vi "SDCP - Standard Message Frames Editor - Load Excel File.vi"(2 "error in (no error)":errorcluster, 3 "Excel File Path":path=path "E:/Projects/System Diagnostics and Control Protocol/SDCP_LabVIEW/Parameter Files/Motion Processing Board - Standard Message Frame List.csv") -> (0 "error out":errorcluster, 1 "Parameters":T2(array[cluster]))   [LabVIEW 2020]
uses:
  Typedefs/SDCP - Standard Message Frames Editor - Parameter cluster.ctl
  <vilib>/Utility/NIReport.llb/Report Type.ctl
  <vilib>/addons/_office/excel.llb/Excel Get Data ([str]).vi
  <vilib>/Utility/NIReport.llb/NI_report.lvclass
  <vilib>/Utility/NIReport.llb/NI_ReportGenerationCore.lvlib
  <vilib>/Utility/NIReport.llb/Excel/NI_Excel.lvclass
  <vilib>/addons/_office/NI_ReportGenerationToolkit.lvlib
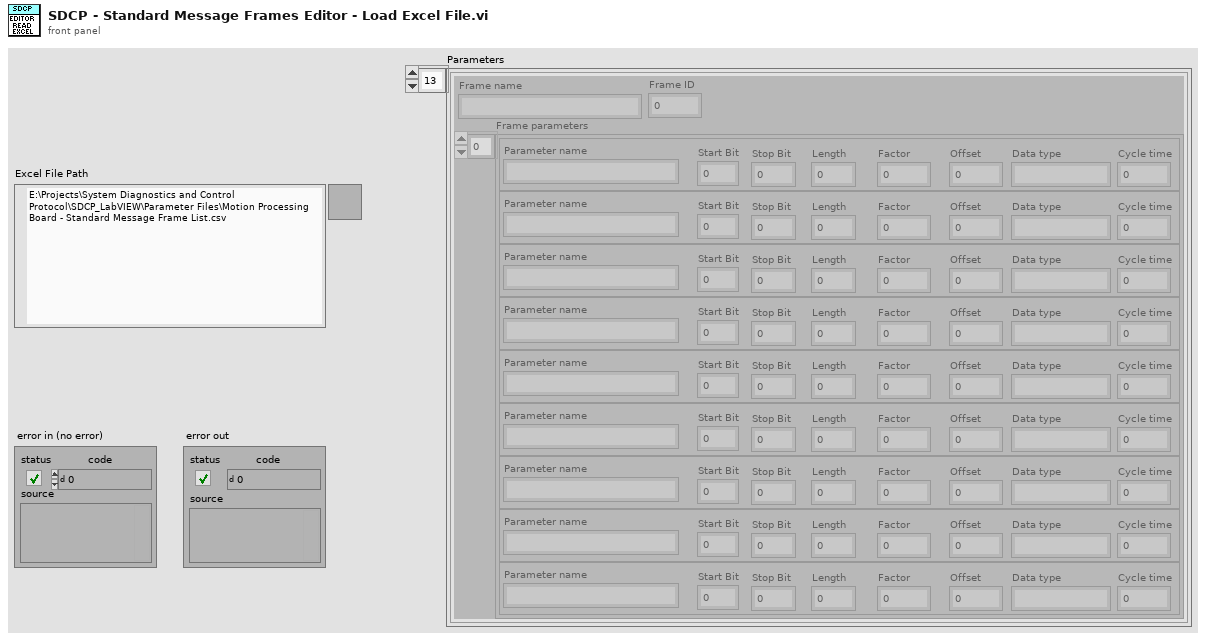
[diagram p1: front panel]
types:
  T1 = typedef "SDCP - Standard Message Frames Editor - Parameter cluster.ctl" = cluster{"Parameter name":string, "Start Bit":i32, "Stop Bit":i32, "Length":i32, "Factor":dbl, "Offset":dbl, "Data type":string, "Cycle time":dbl}
  T2 = cluster{"Frame name":string, "Frame ID":i32, "Frame parameters":T1[]}[]
  T3 = typedef "NI_ReportGenerationCore.lvlib/Report Type.ctl" = enum16{"HTML", "Word", "Excel"}
  T4 = enum16{"maximized", "minimized", "normal", "no change"}
  T5 = cluster{"Frame name":string, "Frame ID":i32, "Frame parameters":T1[]}
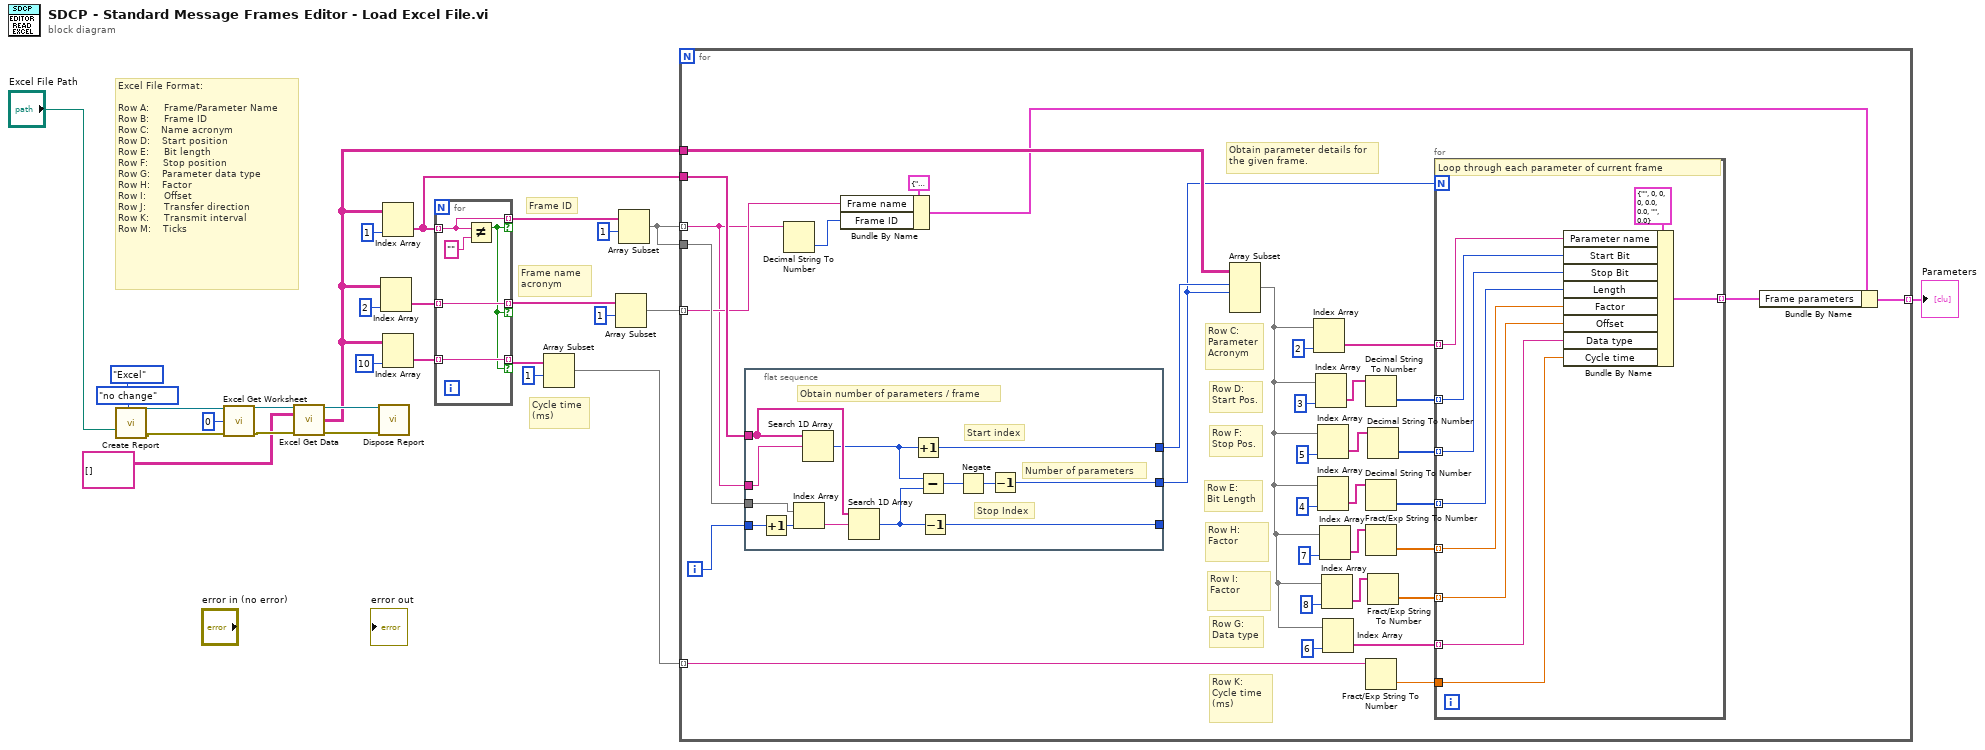
[diagram p0: block diagram]
diagram:
  # "Cycle time\n(ms)"
  # "Frame name \nacronym"
  # "Frame ID"
  # "Excel File Format: \n\nRow A:     Frame/Parameter Name\nRow B:     Frame ID\nRow C:    Name acronym\nRow D:    Start position\nRow E:     Bit length\nRow F:     Stop position\nRow G:    Parameter data type\nRow H:    Factor\nRow I:      Offset\nRow J:      Transfer direction\nRow K:     Transmit interval\nRow M:    Ticks"
  n1 = call <vilib>:"Create Report.vi"("window state (normal)"=T4."no change", "report type"=Report_Type."Excel", "template (empty)"="Excel File Path") -> ("report out"=w24:refnum<class "NI_report.lvclass">, "error out"=w25:errorcluster)  [unwired: 11 in]
  n2 = call <vilib>:"Excel Get Worksheet.vi"("report in"=w24, "worksheet index (0)"=0, "error in (no error)"=w25) -> ("report out"=w22:refnum<class "NI_report.lvclass">, "error out"=w21:errorcluster)  [unwired: 11 in]
  n3 = call-poly <vilib>:"Excel Get Data.vi"("report in"=w22, "data type"=string[][] [], "error in (no error)"=w21) -> ("report out"=w12:refnum<class "NI_report.lvclass">, "data"=w5:string[][], "error out"=w11:errorcluster)  [unwired: 10 in]
  n4 = call-dynamic "Dispose Report.vi"("report in"=w12, "error in (no error)"=w11) -> ()  [unwired: 13 in, 1 out]
  n5 = Index Array(array=w5, index (col)=2 ("disabled index (col)")) -> (element=w15:string[])  [unwired: 1 in]
  n6 = Index Array(array=w5, index (col)=1 ("disabled index (col)")) -> (element=w9:string[])  [unwired: 1 in]
  n7 = Index Array(array=w5, index (col)=10 ("disabled index (col)")) -> (element=w4:string[])  [unwired: 1 in]
  n8 = for {
    tunnel: w9 -> [w32] mode=indexing
    tunnel: [w32] -> w18 mode=indexing if=w29
    tunnel: w15 -> [w31] mode=indexing
    tunnel: [w31] -> w13 mode=indexing if=w29
    tunnel: w4 -> [w30] mode=indexing
    tunnel: [w30] -> w2 mode=indexing if=w29
    n9 = Not Equal?(x=w32, y="") -> (x != y?=w29:bool)
  }
  n10 = Array Subset(array=w2, index=1) -> (w1:string[])  [unwired: 1 in]
  n11 = Array Subset(array=w13, index=1) -> (w10:string[])  [unwired: 1 in]
  n12 = Array Subset(array=w18, index=1) -> (w8:string[])  [unwired: 1 in]
  n13 = for {
    tunnel: w8 -> [w63] mode=indexing
    tunnel: w10 -> [w64] mode=indexing
    tunnel: w5 -> [w61]
    tunnel: w9 -> [w66]
    tunnel: w8 -> [w68]
    tunnel: [w39] -> w7 mode=indexing
    tunnel: w1 -> [w34] mode=indexing
    i -> [w67]
    # "Row G:\nData type"
    # "Row K:\nCycle time\n(ms)"
    # "Row I:\nFactor"
    # "Row H:\nFactor"
    # "Row E:\nBit Length"
    # "Row F: \nStop Pos."
    # "Row D:\nStart Pos."
    # "Row C: \nParameter\nAcronym"
    # "Obtain parameter details for\nthe given frame."
    n14 = flat-sequence {
      tunnel: w63 -> [w91]
      tunnel: w68 -> [w90]
      tunnel: w67 -> [w89]
      tunnel: w66 -> [w87]
      tunnel: [w83] -> w59
      tunnel: [w81] -> w60
      tunnel: [w79] -> _
      frame #0 {
        # "Stop Index"
        # "Number of parameters"
        # "Start index"
        # "Obtain number of parameters / frame"
        n15 = Increment(x=w89) -> (x+1=w88:i32)
        n16 = Index Array(array=w90, index=w88) -> (element=w85:string)
        n17 = Search 1D Array(1D array=w87, element=w91) -> (index of element=w82:i32)  [unwired: 1 in]
        n18 = Search 1D Array(1D array=w87, element=w85) -> (index of element=w80:i32)  [unwired: 1 in]
        n19 = Increment(x=w82) -> (x+1=w81:i32)
        n20 = Subtract(x=w82, y=w80) -> (x-y=w86:i32)
        n21 = Decrement(x=w80) -> (x-1=w79:i32)
        n22 = Negate(x=w86) -> (-x=w84:i32)
        n23 = Decrement(x=w84) -> (x-1=w83:i32)
      }
    }
    n24 = Decimal String To Number(string=w63) -> (number=w62:i32)  [unwired: 2 in, 1 out]
    n25 = Bundle By Name(cluster=T5 {"Frame name"="", "Frame ID"=0, "Frame parameters"=[]}, "Frame name"=w64, "Frame ID"=w62) -> (w41:T5)
    n26 = Array Subset(array=w61, index (row)=w60, length (row)=w59) -> (w36:string[][])  [unwired: 2 in]
    n27 = Index Array(array=w36, index (col)=2 ("disabled index (col)")) -> (element=w57:string[])  [unwired: 1 in]
    n28 = Index Array(array=w36, index (col)=3 ("disabled index (col)")) -> (element=w53:string[])  [unwired: 1 in]
    n29 = Index Array(array=w36, index (col)=5 ("disabled index (col)")) -> (element=w51:string[])  [unwired: 1 in]
    n30 = Index Array(array=w36, index (col)=4 ("disabled index (col)")) -> (element=w49:string[])  [unwired: 1 in]
    n31 = Index Array(array=w36, index (col)=7 ("disabled index (col)")) -> (element=w46:string[])  [unwired: 1 in]
    n32 = Index Array(array=w36, index (col)=8 ("disabled index (col)")) -> (element=w43:string[])  [unwired: 1 in]
    n33 = Index Array(array=w36, index (col)=6 ("disabled index (col)")) -> (element=w35:string[])  [unwired: 1 in]
    n34 = Decimal String To Number(string=w53) -> (number=w52:i32[])  [unwired: 2 in, 1 out]
    n35 = Decimal String To Number(string=w49) -> (number=w48:i32[])  [unwired: 2 in, 1 out]
    n36 = Fract/Exp String To Number(string=w46) -> (number=w45:dbl[])  [unwired: 3 in, 1 out]
    n37 = Fract/Exp String To Number(string=w34) -> (number=w38:dbl)  [unwired: 3 in, 1 out]
    n38 = Decimal String To Number(string=w51) -> (number=w50:i32[])  [unwired: 2 in, 1 out]
    n39 = Fract/Exp String To Number(string=w43) -> (number=w42:dbl[])  [unwired: 3 in, 1 out]
    n40 = for {
      N: w59 -> [_]
      tunnel: w57 -> [w77] mode=indexing
      tunnel: w52 -> [w76] mode=indexing
      tunnel: w50 -> [w75] mode=indexing
      tunnel: w48 -> [w74] mode=indexing
      tunnel: w45 -> [w73] mode=indexing
      tunnel: w42 -> [w72] mode=indexing
      tunnel: [w71] -> w40 mode=indexing
      tunnel: w38 -> [w70]
      tunnel: w35 -> [w69] mode=indexing
      # "Loop through each parameter of current frame"
      n41 = Bundle By Name(cluster=T1 {"Parameter name"="", "Start Bit"=0, "Stop Bit"=0, "Length"=0, "Factor"=0.0, "Offset"=0.0, "Data type"="", "Cycle time"=0.0}, "Parameter name"=w77, "Start Bit"=w76, "Stop Bit"=w75, "Length"=w74, "Factor"=w73, "Offset"=w72, "Data type"=w69, "Cycle time"=w70) -> (w71:T1)
    }
    n42 = Bundle By Name(cluster=w41, "Frame parameters"=w40) -> (w39:T5)
  }
  "Parameters" <- w7
